vi "LinuxLigixúc.vi"() -> ()   [LabVIEW 2018]
panel:
  out "x .or. y?":u8
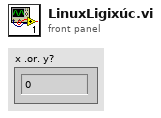
[diagram p1: front panel]
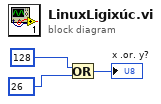
[diagram p0: block diagram]
diagram:
  n1 = Or(x=u8 128, y=u8 26) -> (x .or. y?=→"x .or. y?":u8)
